vi "LogFrequencyDomainData.vi"(0 "Logging Configuration Input":T3, 1 "Data Notifier":refnum<notifier>, 5 "QueuedDataInput":T1, 11 "error in (no error)":errorcluster) -> (4 "Logging Configuration Output":T3, 15 "error out":errorcluster)   [LabVIEW 2022 SP3, in "Logging.lvlib"]
doc: "Use the Write To Measurement File Express VI to log data to disk in a LVM file."
uses:
  Logging.lvlib
  Logging Configuration.ctl
  support/TDMS-Refs.ctl
  QueuedLoggedData.ctl
  FFT-Data.ctl
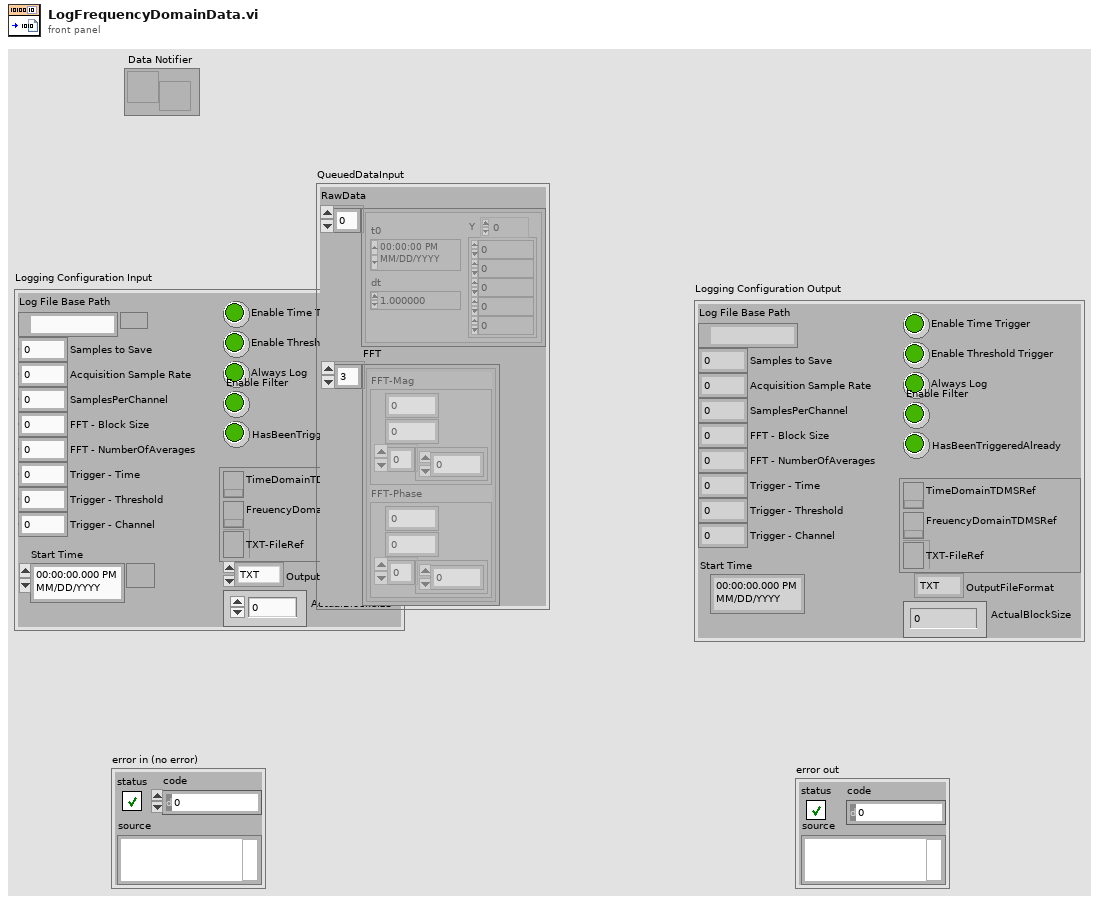
[diagram p1: front panel]
types:
  T1 = typedef "QueuedLoggedData.ctl" = cluster{"RawData":waveform(dbl)[], "FFT ":T2[]}
  T2 = typedef "FFT-Data.ctl" = cluster{"FFT-Mag":cluster{"t0":dbl, "dt":dbl, "Y":dbl[]}, "FFT-Phase":cluster{"t0":dbl, "dt":dbl, "Y":dbl[]}}
  T3 = typedef "Logging.lvlib/Logging Configuration.ctl" = cluster{"Log File Base Path":path, "Samples to Save":u32, "Acquisition Sample Rate":dbl, "SamplesPerChannel":u32, "FFT - Block Size":u32, "FFT - NumberOfAverages":i32, "Trigger - Time":i32, "Trigger - Threshold":dbl, "Trigger - Channel":u32, "Enable Time Trigger":bool, "Enable Threshold Trigger":bool, "Always Log":bool, "Enable Filter":bool, "FilesRefs":T4, "OutputFileFormat":enum16{"TXT", "TDMS"}, "ActualBlockSize":i32, "HasBeenTriggeredAlready":bool, "Start Time":timestamp}
  T4 = typedef "TDMS-Refs.ctl" = cluster{"TimeDomainTDMSRef":refnum<k34>, "FreuencyDomainTDMSRef":refnum<k34>, "TXT-FileRef":refnum<file>}
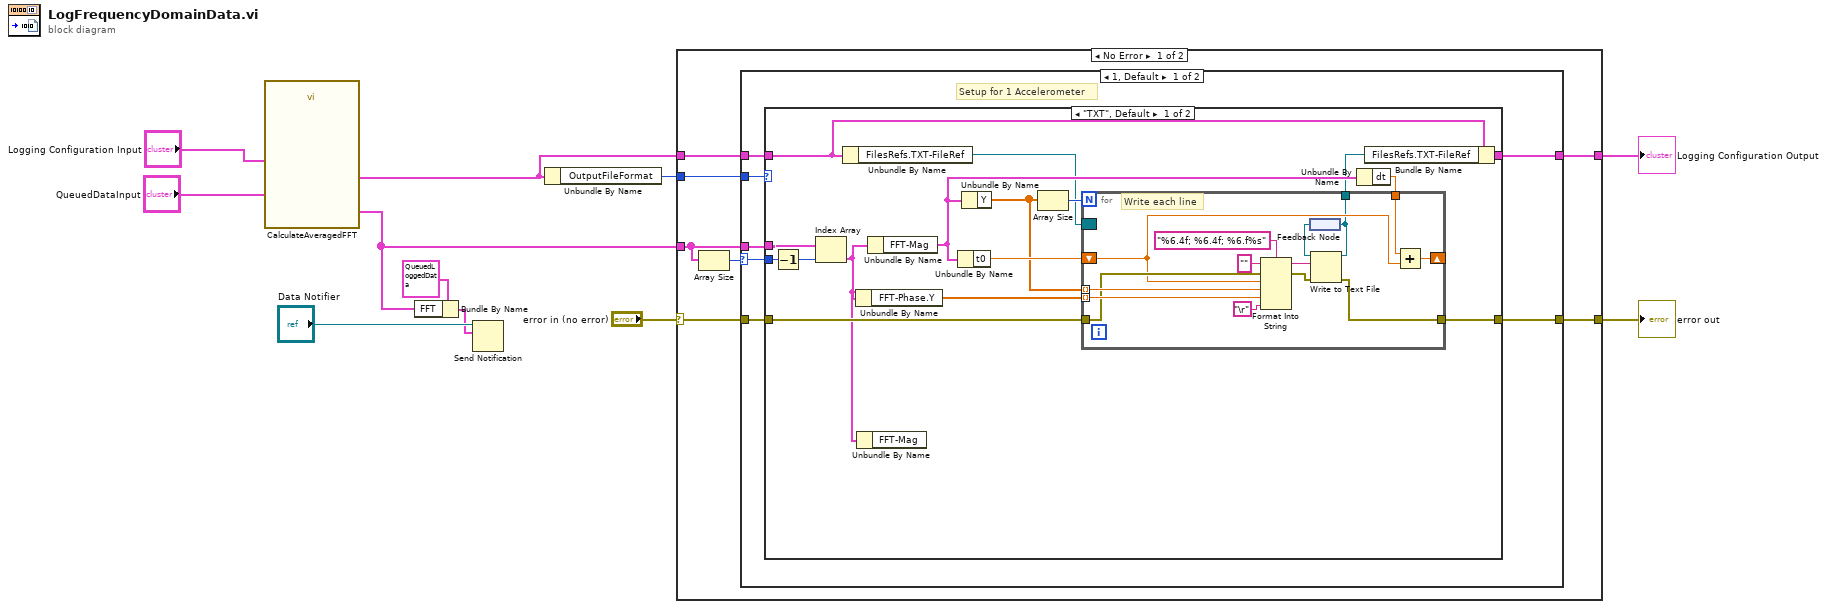
[diagram p0: block diagram]
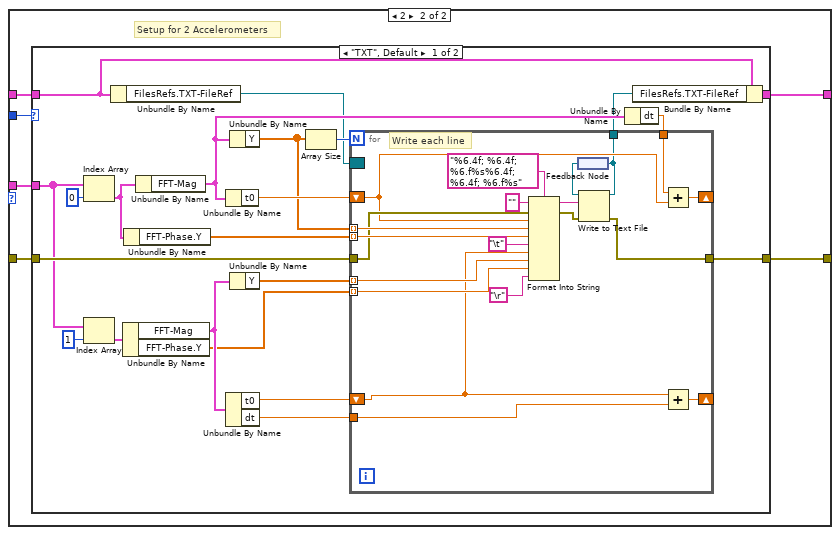
[diagram p3: hidden frame]
diagram:
  n1 = call "CalculateAveragedFFT.vi"("QueuedDataInput"="QueuedDataInput", "Logging Settings Input"="Logging Configuration Input") -> ("FFT Cluster Output"=w2:T2[], "Logging Settings Output"=w6:T3)  [unwired: 4 in]
  n2 = Bundle By Name(cluster=T1 {"RawData"=[{"t0"=timestamp(3776456435.5591307 s since 1904-01-01), "dt"=6.103515510305635e-05, "Y"=array[1638 elements], "attributes"=variant("NI_ChannelName"=variant(string "Accel-ai0"), "NI_UnitDescription"=variant(string "m/s^2"), "NI_dBReference"=variant(dbl 1.0))}, {"t0"=timestamp(3776456435.5591307 s since 1904-01-01), "dt"=6.103515510305635e-05, "Y"=array[1638 elements], "attributes"=variant("NI_ChannelName"=variant(string "Accel-ai1"), "NI_UnitDescription"=variant(string "m/s^2"), "NI_dBReference"=variant(dbl 1.0))}], "FFT "=[]} ("QueuedDataInput"), "FFT"=w2) -> (w1:T1)
  n3 = Send Notification(notification=w1, notifier="Data Notifier") -> ()  [unwired: 1 in, 2 out]
  n4 = Unbundle By Name(w6) -> ("OutputFileFormat"=w9:enum16{"TXT", "TDMS"})
  n5 = case shown="No Error" "error in (no error)" {
    selector: "error in (no error)" -> [w16 w109]
    tunnel: w6 -> [w18 w108]
    tunnel: [w17 w109] -> w11
    tunnel: w9 -> [w15 _]
    tunnel: w2 -> [w12 _]
    tunnel: [w14 w108] -> w8
    frame No Error {
      n6 = Array Size(array=w12) -> (size(s)=w13:i32)
      n7 = case shown="1, Default" w13 {
        selector: w13 -> [w19 _]
        tunnel: w18 -> [w25 w63]
        tunnel: [w24 w62] -> w17
        tunnel: w16 -> [w23 w61]
        tunnel: w15 -> [w22 w60]
        tunnel: w12 -> [w21 w59]
        tunnel: [w20 w58] -> w14
        frame 1, Default {
          # "Setup for 1 Accelerometer"
          n8 = case shown="\"TXT\", Default" w22 {
            tunnel: w25 -> [w33 w57]
            tunnel: [w36 w56] -> w24
            tunnel: w23 -> [w37 w56]
            tunnel: w21 -> [w29 _]
            tunnel: [w32 w57] -> w20
            tunnel: w19 -> [w28 _]
            frame "TXT", Default {
              n9 = Decrement(x=w28) -> (x-1=w27:i32)
              n10 = Index Array(array=w29, index=w27) -> (element=w26:T2)
              n11 = Unbundle By Name(w33) -> ("FilesRefs.TXT-FileRef"=w31:refnum<file>)
              n12 = Unbundle By Name(w26) -> ("FFT-Phase.Y"=w38:dbl[])
              n13 = Unbundle By Name(w26) -> ()  [unwired: 1 out]
              n14 = Unbundle By Name(w26) -> ("FFT-Mag"=w35:cluster{"t0":dbl, "dt":dbl, "Y":dbl[]})
              n15 = Unbundle By Name(w35) -> ("t0"=w40:dbl)
              n16 = Unbundle By Name(w35) -> ("Y"=w39:dbl[])
              n17 = Array Size(array=w39) -> (size(s)=w41:i32)
              n18 = Unbundle By Name(w35) -> ("dt"=w34:dbl)
              n19 = for {
                N: w41 -> [_]
                tunnel: w39 -> [w53] mode=indexing
                shift-right: [w50] -> _
                shift-left: w40 -> [w48]
                tunnel: w38 -> [w52] mode=indexing
                tunnel: w37 -> [w51]
                tunnel: [w45] -> w36
                tunnel: w34 -> [w49]
                border: w31 -> [_]
                tunnel: [w43] -> w30
                # "Write each line"
                n20 = Format Into String(format string="%6.4f; %6.4f; %6.f%s", initial string="", error in=w51, w48, w53, w52, "\r") -> (resulting string=w47:string, error out=w46:errorcluster)
                n21 = feedback #1() -> (w44:refnum<file>)
                n22 = Write to Text File(file (use dialog)=w44, text=w47, error in=w46) -> (refnum out=w43:refnum<file>, error out=w45:errorcluster)  [unwired: 1 in, 1 out]
                n23 = feedback-in #1(w43) -> ()
                n24 = Add(x=w49, y=w48) -> (x+y=w50:dbl)
              }
              n25 = Bundle By Name(cluster=w33, "FilesRefs.TXT-FileRef"=w30) -> (w32:T3)
            }
            frame "TDMS" {
            }
          }
        }
        frame 2 {
          # "Setup for 2 Accelerometers"
          n26 = case shown="\"TXT\", Default" w60 {
            tunnel: w63 -> [w77 w107]
            tunnel: [w80 w106] -> w62
            tunnel: w61 -> [w81 w106]
            tunnel: w59 -> [w68 _]
            tunnel: [w76 w107] -> w58
            frame "TXT", Default {
              n27 = Index Array(array=w68, index=0) -> (element=w73:T2)
              n28 = Index Array(array=w68, index=1) -> (element=w70:T2)
              n29 = Unbundle By Name(w77) -> ("FilesRefs.TXT-FileRef"=w75:refnum<file>)
              n30 = Unbundle By Name(w70) -> ("FFT-Mag"=w71:cluster{"t0":dbl, "dt":dbl, "Y":dbl[]}, "FFT-Phase.Y"=w66:dbl[])
              n31 = Unbundle By Name(w73) -> ("FFT-Phase.Y"=w82:dbl[])
              n32 = Unbundle By Name(w73) -> ("FFT-Mag"=w79:cluster{"t0":dbl, "dt":dbl, "Y":dbl[]})
              n33 = Unbundle By Name(w79) -> ("t0"=w84:dbl)
              n34 = Unbundle By Name(w71) -> ("t0"=w65:dbl, "dt"=w64:dbl)
              n35 = Unbundle By Name(w79) -> ("Y"=w83:dbl[])
              n36 = Unbundle By Name(w71) -> ("Y"=w69:dbl[])
              n37 = Array Size(array=w83) -> (size(s)=w85:i32)
              n38 = Unbundle By Name(w79) -> ("dt"=w78:dbl)
              n39 = for {
                N: w85 -> [_]
                tunnel: w83 -> [w103] mode=indexing
                shift-right: [w100] -> _
                shift-left: w84 -> [w98]
                tunnel: w82 -> [w102] mode=indexing
                tunnel: w81 -> [w101]
                tunnel: [w95] -> w80
                tunnel: w78 -> [w99]
                border: w75 -> [_]
                tunnel: [w93] -> w74
                tunnel: w69 -> [w90] mode=indexing
                tunnel: w66 -> [w89] mode=indexing
                shift-right: [w88] -> _
                shift-left: w65 -> [w86]
                tunnel: w64 -> [w87]
                # "Write each line"
                n40 = Format Into String(format string="%6.4f; %6.4f; %6.f%s%6.4f; %6.4f; %6.f%s", initial string="", error in=w101, w98, w103, w102, "\t", w86, w90, w89, "\r") -> (resulting string=w97:string, error out=w96:errorcluster)
                n41 = feedback #2() -> (w94:refnum<file>)
                n42 = Write to Text File(file (use dialog)=w94, text=w97, error in=w96) -> (refnum out=w93:refnum<file>, error out=w95:errorcluster)  [unwired: 1 in, 1 out]
                n43 = feedback-in #2(w93) -> ()
                n44 = Add(x=w99, y=w98) -> (x+y=w100:dbl)
                n45 = Add(x=w86, y=w87) -> (x+y=w88:dbl)
              }
              n46 = Bundle By Name(cluster=w77, "FilesRefs.TXT-FileRef"=w74) -> (w76:T3)
            }
            frame "TDMS" {
            }
          }
        }
      }
    }
    frame Error {
    }
  }
  "error out" <- w11
  "Logging Configuration Output" <- w8
